vi "Is Created Queue.vi"(7 "jettl in":refnum<class "jettl.lvclass">, 9 "Created Queue Alias":string, 10 "Queue Mailbox":refnum<data-value>) -> (2 "Is Created Queue?":bool, 5 "jettl out":refnum<class "jettl.lvclass">)   [LabVIEW 2021, in "jettl.lvlib" / "Queue Mailbox.lvlib"]
uses:
  Queue Mailbox.lvlib
  jettl/jettl.lvclass
  Queue Mailbox/Queue Mailbox.lvclass
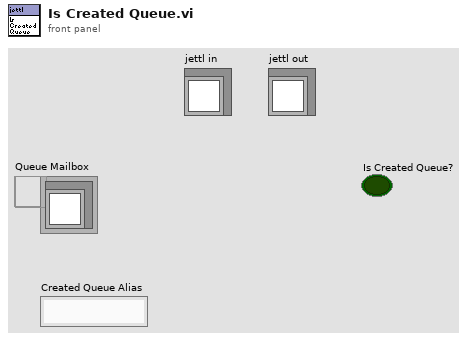
[diagram p1: front panel]
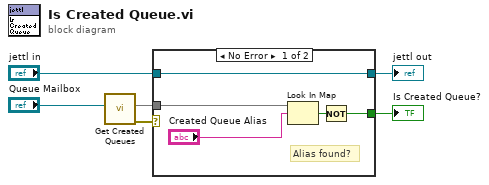
[diagram p0: block diagram]
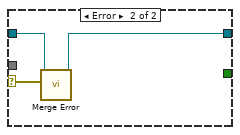
[diagram p2: hidden frame]
diagram:
  n1 = call "Get Created Queues.vi"("Queue Mailbox"="Queue Mailbox") -> ("error out"=w5:errorcluster, "Created Queues"=w2:map{string, refnum<data-value>})  [unwired: 9 in]
  n2 = case shown="No Error" w5 {
    selector: w5 -> [_ w12]
    tunnel: [w11 w13] -> w3
    tunnel: "jettl in" -> [w11 w14]
    tunnel: w2 -> [w8 _]
    tunnel: [w7 _] -> w1
    frame No Error {
      # "Alias found?"
      n3 = Look In Map(map=w8, key="Created Queue Alias") -> (key not found?=w9:bool)  [unwired: 1 in, 1 out]
      n4 = Not(x=w9) -> (.not. x?=w7:bool)
    }
    frame Error {
      n5 = call-dynamic "Merge Error.vi"("Error"=w12, "Merge Error in"=w14) -> ("Merge Error out"=w13:refnum<class "jettl.lvclass">)  [unwired: 9 in]
    }
  }
  "jettl out" <- w3
  "Is Created Queue?" <- w1
